vi "ADB log catch.vi"() -> ()   [LabVIEW 2023]
panel:
  out "number":i32
  out "after substring":string
  out "before substring":string
  out "error out":errorcluster
  out "standard output":string
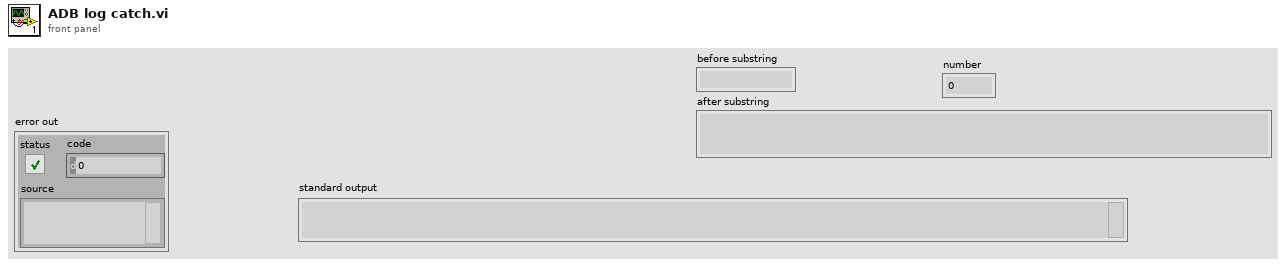
[diagram p1: front panel]
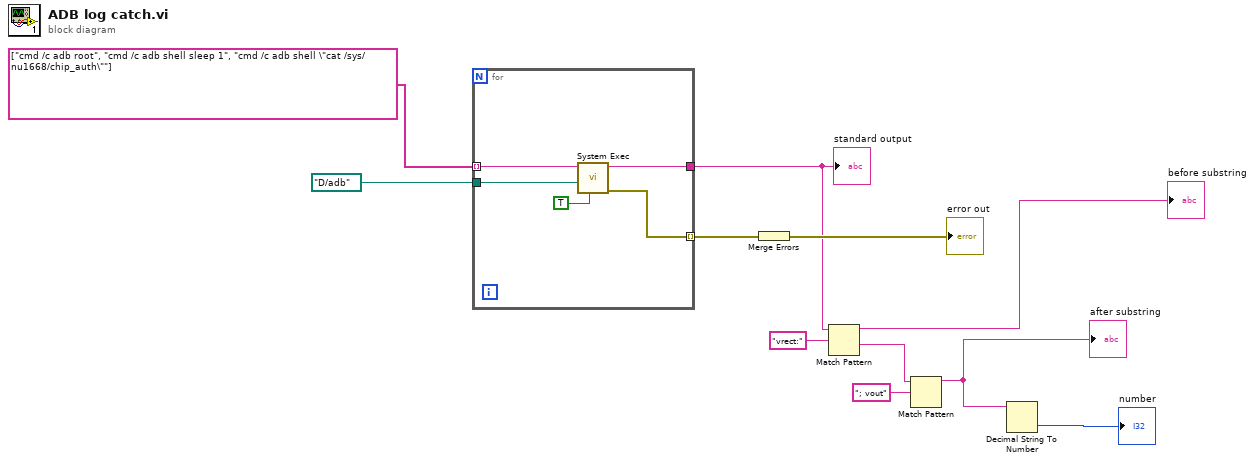
[diagram p0: block diagram]
diagram:
  n1 = for {
    tunnel: path "D:/adb" ("working directory") -> [w16]
    tunnel: string[] ["cmd /c adb root", "cmd /c adb shell sleep 1", "cmd /c adb shell \"cat /sys/nu1668/chip_auth\""] -> [w15] mode=indexing
    tunnel: [w14] -> w7
    tunnel: [w13] -> w9 mode=indexing
    n2 = call <vilib>:"System Exec.vi"("run minimized? (F)"=TRUE, "working directory"=w16, "command line"=w15) -> ("error out"=w13:errorcluster, "standard output"=w14:string)  [unwired: 5 in, 2 out]
  }
  "standard output" <- w7
  n3 = Merge Errors(w9) -> (→"error out":errorcluster)
  n4 = Match Pattern(string=w7, regular expression="vrect:") -> (before substring=→"before substring":string, after substring=w4:string)  [unwired: 1 in, 2 out]
  n5 = Match Pattern(string=w4, regular expression="; vout") -> (before substring=w2:string)  [unwired: 1 in, 3 out]
  "after substring" <- w2
  n6 = Decimal String To Number(string=w2) -> (number=→"number":i32)  [unwired: 2 in, 1 out]
